vi "VISA01_serial01_Open.vi"(11 "YTESTER测试数据":T1 caption="不要修改！") -> (3 "YTESTER结论":T2)   [LabVIEW 2017]
uses:
  YtCommon.lvlibp/yt`Step StepBaseInput.ctl
  YtCommon.lvlibp/yt`Step StepResult.ctl
  YtCommon.lvlibp/yt`Step TestData.ctl
  YtCommon.lvlibp/yt`Step System Queue.ctl
  58f0560a-0019-436e-a3dd-a0b864a05705.vi
  <vilib>/Instr/_visa.llb/VISA Configure Serial Port (Instr).vi
  YtCommon.lvlibp
panel:
  in  "YTESTER开放参数":T4={"YTESTER_BaseInput"={"isTest"=TRUE, "isSkip"=FALSE, "StepName"="VISA打开", "OnPass"=enum."Next", "OnFail"=enum."Terminate", "ReTestNumber"=0.0}, "VISA resource"="", "baud rate (9600)"="9600", "termination char(0xA = '\\n' = LF) "=10, "timeout (3sec)"=3000, "Enable Termination Char (F)"=FALSE, "flow control (0:none)"=0, "data bits (8)"=8, "parity (0:none)"=enum."None", "stop bits (10: 1 bit)"=enum."1.0"} {"data bits (8)" min=5 max=8 step=1; "flow control (0:none)" items=["None", "XON/XOFF", "RTS/CTS", "XON/XOFF & RTS/CTS", "DTR/DSR", "XON/XOFF & DTR/DSR"]; "termination char(0xA = '\\n' = LF)" format="%.0x"}
  # "串口打开\nVISA OPEN"
  # "重入！"
  # "YYLL修改了紫色区域默认值"
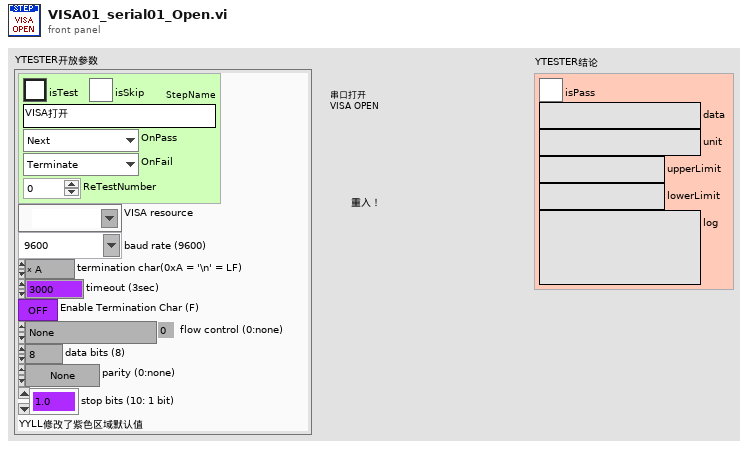
[diagram p1: front panel]
types:
  T1 = typedef "YtCommon.lvlibp/yt`Step TestData.ctl" = cluster{"Socket(From1)":i32, "SN":refnum<notifier>, "StopFlagRef":refnum<notifier>, "YT System Queue":refnum<queue>}
  T2 = typedef "YtCommon.lvlibp/yt`Step StepResult.ctl" = cluster{"isPass":bool, "data":string, "unit":string, "upperLimit":string, "lowerLimit":string, "log":string}
  T3 = typedef "YtCommon.lvlibp/yt`Step StepBaseInput.ctl" = cluster{"isTest":bool, "isSkip":bool, "StepName":string, "OnPass":enum16{"Next", "ToOVER", "Terminate"}, "OnFail":enum16{"Next", "ToOVER", "Terminate"}, "ReTestNumber":dbl}
  T4 = cluster{"YTESTER_BaseInput":T3, "VISA resource":refnum<visa-resource-name>, "baud rate (9600)":string, "termination char(0xA = '\\n' = LF) ":u8, "timeout (3sec)":u32, "Enable Termination Char (F)":bool, "flow control (0:none)":u16, "data bits (8)":u16, "parity (0:none)":enum16{"None", "Odd", "Even", "Mark", "Space"}, "stop bits (10: 1 bit)":enum16{"1.0", "1.5", "2.0"}}
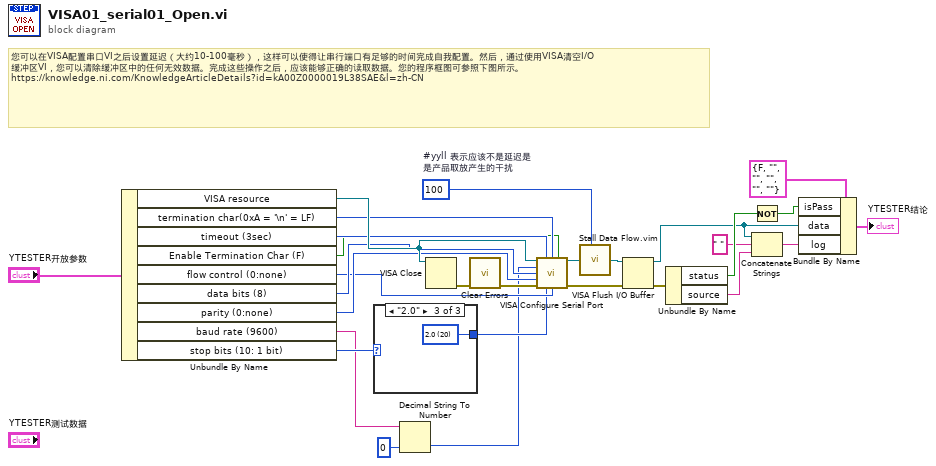
[diagram p0: block diagram]
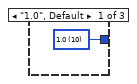
[diagram p2: hidden frame]
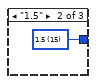
[diagram p3: hidden frame]
diagram:
  w6 = u32 100  # #yyll 表示应该不是延迟是 是产品取放产生的干扰
  # "您可以在VISA配置串口VI之后设置延迟（大约10-100毫秒），这样可以使得让串行端口有足够的时间完成自我配置。然后，通过使用VISA清空I/O 缓冲区VI，您可以清除缓冲区中的任何无效数据。完成这些操作之后，应该能够正确的读取数据。您的程序框图可参照下图所示。\nhttps://knowledge.ni.com/KnowledgeArticleDetails?id=kA00Z0000019L38SAE&l=zh-CN"
  n1 = Unbundle By Name("YTESTER开放参数") -> ("VISA resource"=w23:refnum<visa-resource-name>, "termination char(0xA = '\\n' = LF)"=w20:u8, "timeout (3sec)"=w21:u32, "Enable Termination Char (F)"=w19:bool, "flow control (0:none)"=w16:u16, "data bits (8)"=w18:u16, "parity (0:none)"=w17:enum16{"None", "Odd", "Even", "Mark", "Space"}, "baud rate (9600)"=w3:string, "stop bits (10: 1 bit)"=w11:enum16{"1.0", "1.5", "2.0"})
  n2 = case shown="\"2.0\"" w11 {
    tunnel: [w29 w30 w31] -> w10
    frame "1.0", Default {
      w29 = u16 10 items=["1.0"=10, "1.5"=15, "2.0"=20] ("stop bits (10: 1 bit)")
    }
    frame "1.5" {
      w30 = u16 15 items=["1.0"=10, "1.5"=15, "2.0"=20] ("stop bits (10: 1 bit)")
    }
    frame "2.0" {
      w31 = u16 20 items=["1.0"=10, "1.5"=15, "2.0"=20] ("stop bits (10: 1 bit)")
    }
  }
  n3 = Decimal String To Number(string=w3, default (0L)=u32 0 ("default (0 I32)")) -> (number=w1:u32)  [unwired: 1 in, 1 out]
  n4 = VISA Close(VISA resource name=w23) -> (error out=w22:errorcluster)  [unwired: 1 in]
  n5 = call <vilib>:"Clear Errors.vi"("error in (no error)"=w22) -> ("error out"=w12:errorcluster)  [unwired: 5 in, 1 out]
  n6 = call-poly "VISA Configure Serial Port"("VISA resource name"=w23, "timeout (10sec)"=w21, "termination char\n(0xA = '\\n' = LF)"=w20, "Enable Termination\nChar (T)"=w19, "baud rate (9600)"=w1, "data bits (8)"=w18, "parity (0:none)"=w17, "error in (no error)"=w12, "stop bits (10: 1 bit)"=w10, "flow control (0:none)"=w16) -> ("VISA resource name out"=w25:refnum<visa-resource-name>, "error out"=w24:errorcluster)  [unwired: 4 in]
  n7 = call "Stall Data Flow.vim"("value in"=w25, "milliseconds to wait"=w6) -> ("value out"=w7:refnum<visa-resource-name>)  [unwired: 1 out]
  n8 = VISA Flush I/O Buffer(VISA resource name=w7, error in (no error)=w24) -> (VISA resource name out=w9:refnum<visa-resource-name>, error out=w15:errorcluster)  [unwired: 1 in]
  n9 = Unbundle By Name(w15) -> ("status"=w14:bool, "source"=w8:string)
  n10 = Not(x=w14) -> (.not. x?=w13:bool)
  n11 = Concatenate Strings(w9, " " ("string"), w8) -> (w5:string)
  n12 = Bundle By Name(cluster=T2 {"isPass"=FALSE, "data"="", "unit"="", "upperLimit"="", "lowerLimit"="", "log"=""} ("Result"), "isPass"=w13, "data"=w9, "log"=w5) -> (→"YTESTER结论":T2)
